vi "Calc - Rho_air.vi"(7 "TPT":dbl, 10 "AIN":dbl, 11 "00-01-9220":dbl[](array[numeric])) -> (1 "MDOT":dbl, 2 "VIN":dbl, 3 "Rho_air":dbl)   [LabVIEW 2018, in "Controller (Host).lvlib"]
uses:
  Controller (Host).lvlib
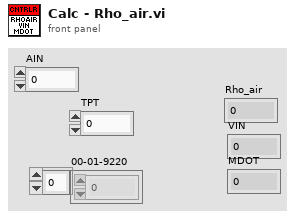
[diagram p1: front panel]
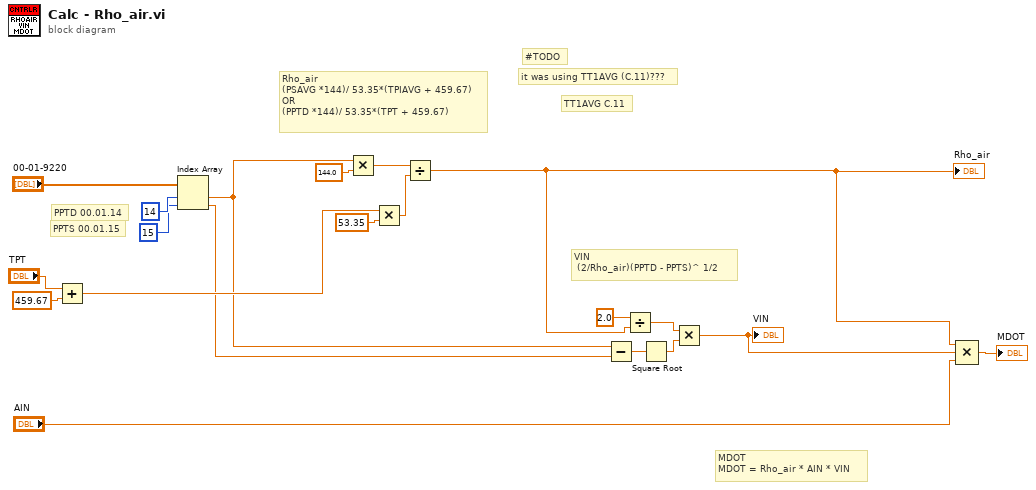
[diagram p0: block diagram]
diagram:
  # "PPTD 00.01.14"
  # "Rho_air\n(PSAVG *144)/ 53.35*(TPIAVG + 459.67)\nOR\n(PPTD *144)/ 53.35*(TPT + 459.67)"
  # "MDOT\nMDOT = Rho_air * AIN * VIN"
  # "PPTS 00.01.15"
  # "VIN\n (2/Rho_air)(PPTD - PPTS)^ 1/2"
  # "#TODO"
  # "it was using TT1AVG (C.11)???"
  # "TT1AVG C.11"
  n1 = Add(x="TPT", y=459.67) -> (x+y=w16:dbl)
  n2 = Index Array(array="00-01-9220", index #1=14 ("index"), index #2=15 ("index")) -> (element #1=w6:dbl, element #2=w5:dbl)
  n3 = Multiply(x=w6, y=144.0) -> (x*y=w15:dbl)
  n4 = Multiply(x=w16, y=53.35) -> (x*y=w17:dbl)
  n5 = Divide(x=w15, y=w17) -> (x/y=w4:dbl)
  "Rho_air" <- w4
  n6 = Subtract(x=w6, y=w5) -> (x-y=w11:dbl)
  n7 = Divide(x=2.0, y=w4) -> (x/y=w9:dbl)
  n8 = Square Root(x=w11) -> (sqrt(x)=w10:dbl)
  n9 = Multiply(x=w9, y=w10) -> (x*y=w3:dbl)
  "VIN" <- w3
  n10 = Compound Arithmetic op=MULTIPLY(w4, w3, "AIN") -> (→"MDOT":dbl)
